vi "Autonomous Independent.vi"() -> ()   [LabVIEW 2012]
doc: "This VI is called when autonomous begins, and will automatically be terminated when autonomous ends. You can carry out timed or sensor driven robot movement independently without needing to return to the caller."
uses:
  Robot Global Data.vi
  Motors Values.vi
panel:
  out "Current Movement, for debugging":T1 {"Y Joystick Value" scale=1.0..-1.0; "X Joystick Value" scale=-1.0..1.0}
  in  "Array of robot movements":T2(array[cluster]) {"Y Joystick Value" scale=1.0..-1.0; "X Joystick Value" scale=-1.0..1.0}
  # "Be sure to right-click and choose Data Operations>>Make Current Value default if you want to save the array values with the VI"
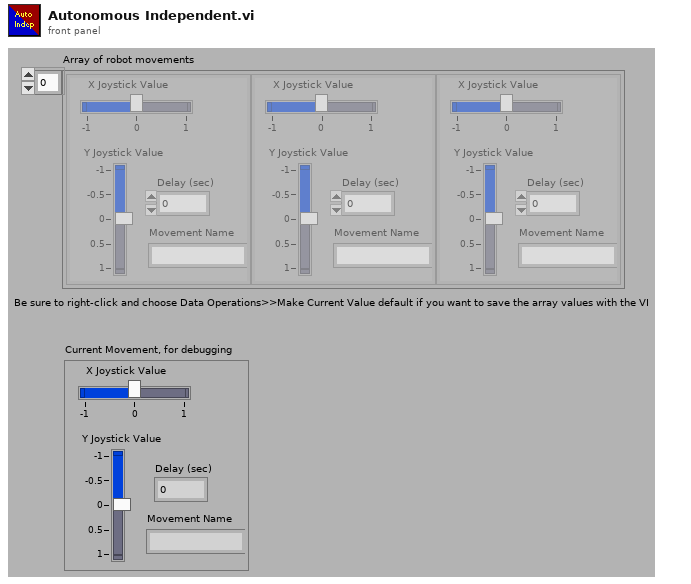
[diagram p1: front panel]
types:
  T1 = cluster{"X Joystick Value":dbl, "Y Joystick Value":dbl, "Delay (sec)":dbl, "Movement Name":string}
  T2 = cluster{"X Joystick Value":dbl, "Y Joystick Value":dbl, "Delay (sec)":dbl, "Movement Name":string}[]
  T3 = typedef "WPI_JoystickDevRef.ctl" = cluster{"Device":T4}
  T4 = typedef "WPI_JoystickDeviceEnum.ctl" = enum16{"USB 1", "USB 2", "USB 3", "USB 4", "Kinect 1", "Kinect 2"}
  T5 = typedef "WPI_DigitalInputDevRef.ctl" = cluster{"DevStatus":errorcluster, "DIO Channel":T6, "Digital Module":T7}
  T6 = typedef "FPGA_DIOChannel.ctl" = enum8{"DIO 1", "DIO 2", "DIO 3", "DIO 4", "DIO 5", "DIO 6", "DIO 7", "DIO 8", "DIO 9", "DIO 10", "DIO 11", "DIO 12", "DIO 13", "DIO 14", "Invalid"}
  T7 = typedef "FPGA_TypedefDigitalModule.ctl" = enum16{"Digital Module 1", "Digital Module 2"}
  T8 = typedef "WPI_RobotDriveDevRef.ctl" = cluster{"DevStatus":errorcluster, "Motors[]":T9[], "Square Inputs":bool, "Max Output":dbl, "Isochronous":bool}
  T9 = typedef "WPI_MotorControlDeviceRef.ctl" = cluster{"DeviceStatus":errorcluster, "Type":enum16{"PWM", "CAN"}, "PWM":cluster{"Digital Module":T7, "PWM Channel":T10, "DeadBand":T11}, "CAN":cluster{"Device Number":u8, "Control Mode":T12, "Semaphore":T13, "Max Vout":dbl}, "Invert":bool, "TransformRef":T14, "InvTransformRef":T14}
  T10 = typedef "FPGA_DIOPWMChannel.ctl" = enum8{"PWM 1", "PWM 2", "PWM 3", "PWM 4", "PWM 5", "PWM 6", "PWM 7", "PWM 8", "PWM 9", "PWM 10", "Invalid"}
  T11 = typedef "WPI_PWMDeadband.ctl" = cluster{"Name":string, "maxPositivePwm":i32, "minPositivePwm":i32, "centerPwm":i32, "maxNegativePwm":i32, "minNegativePwm":i32, "angularRange":u16}
  T12 = typedef "WPI_CANJaguar_ControlMode.ctl" = enum8{"Percent VBus", "Current", "Speed", "Position", "Voltage"}
  T13 = typedef "Semaphore RefNum" = refnum<k1>
  T14 = typedef "WPI_PWMTransform_ConPane.ctl" = refnum<vi>
  T15 = typedef "WPI_ServoDeviceRef.ctl" = cluster{"DeviceStatus":errorcluster, "Digital Module":T7, "PWM Channel":T10, "DeadBand":T11}
  T16 = cluster{"axis 1 (x)":dbl, "axis 2 (y)":dbl, "axis 3 (throttle)":dbl, "axis 4":dbl, "axis 5":dbl, "axis 6":dbl}
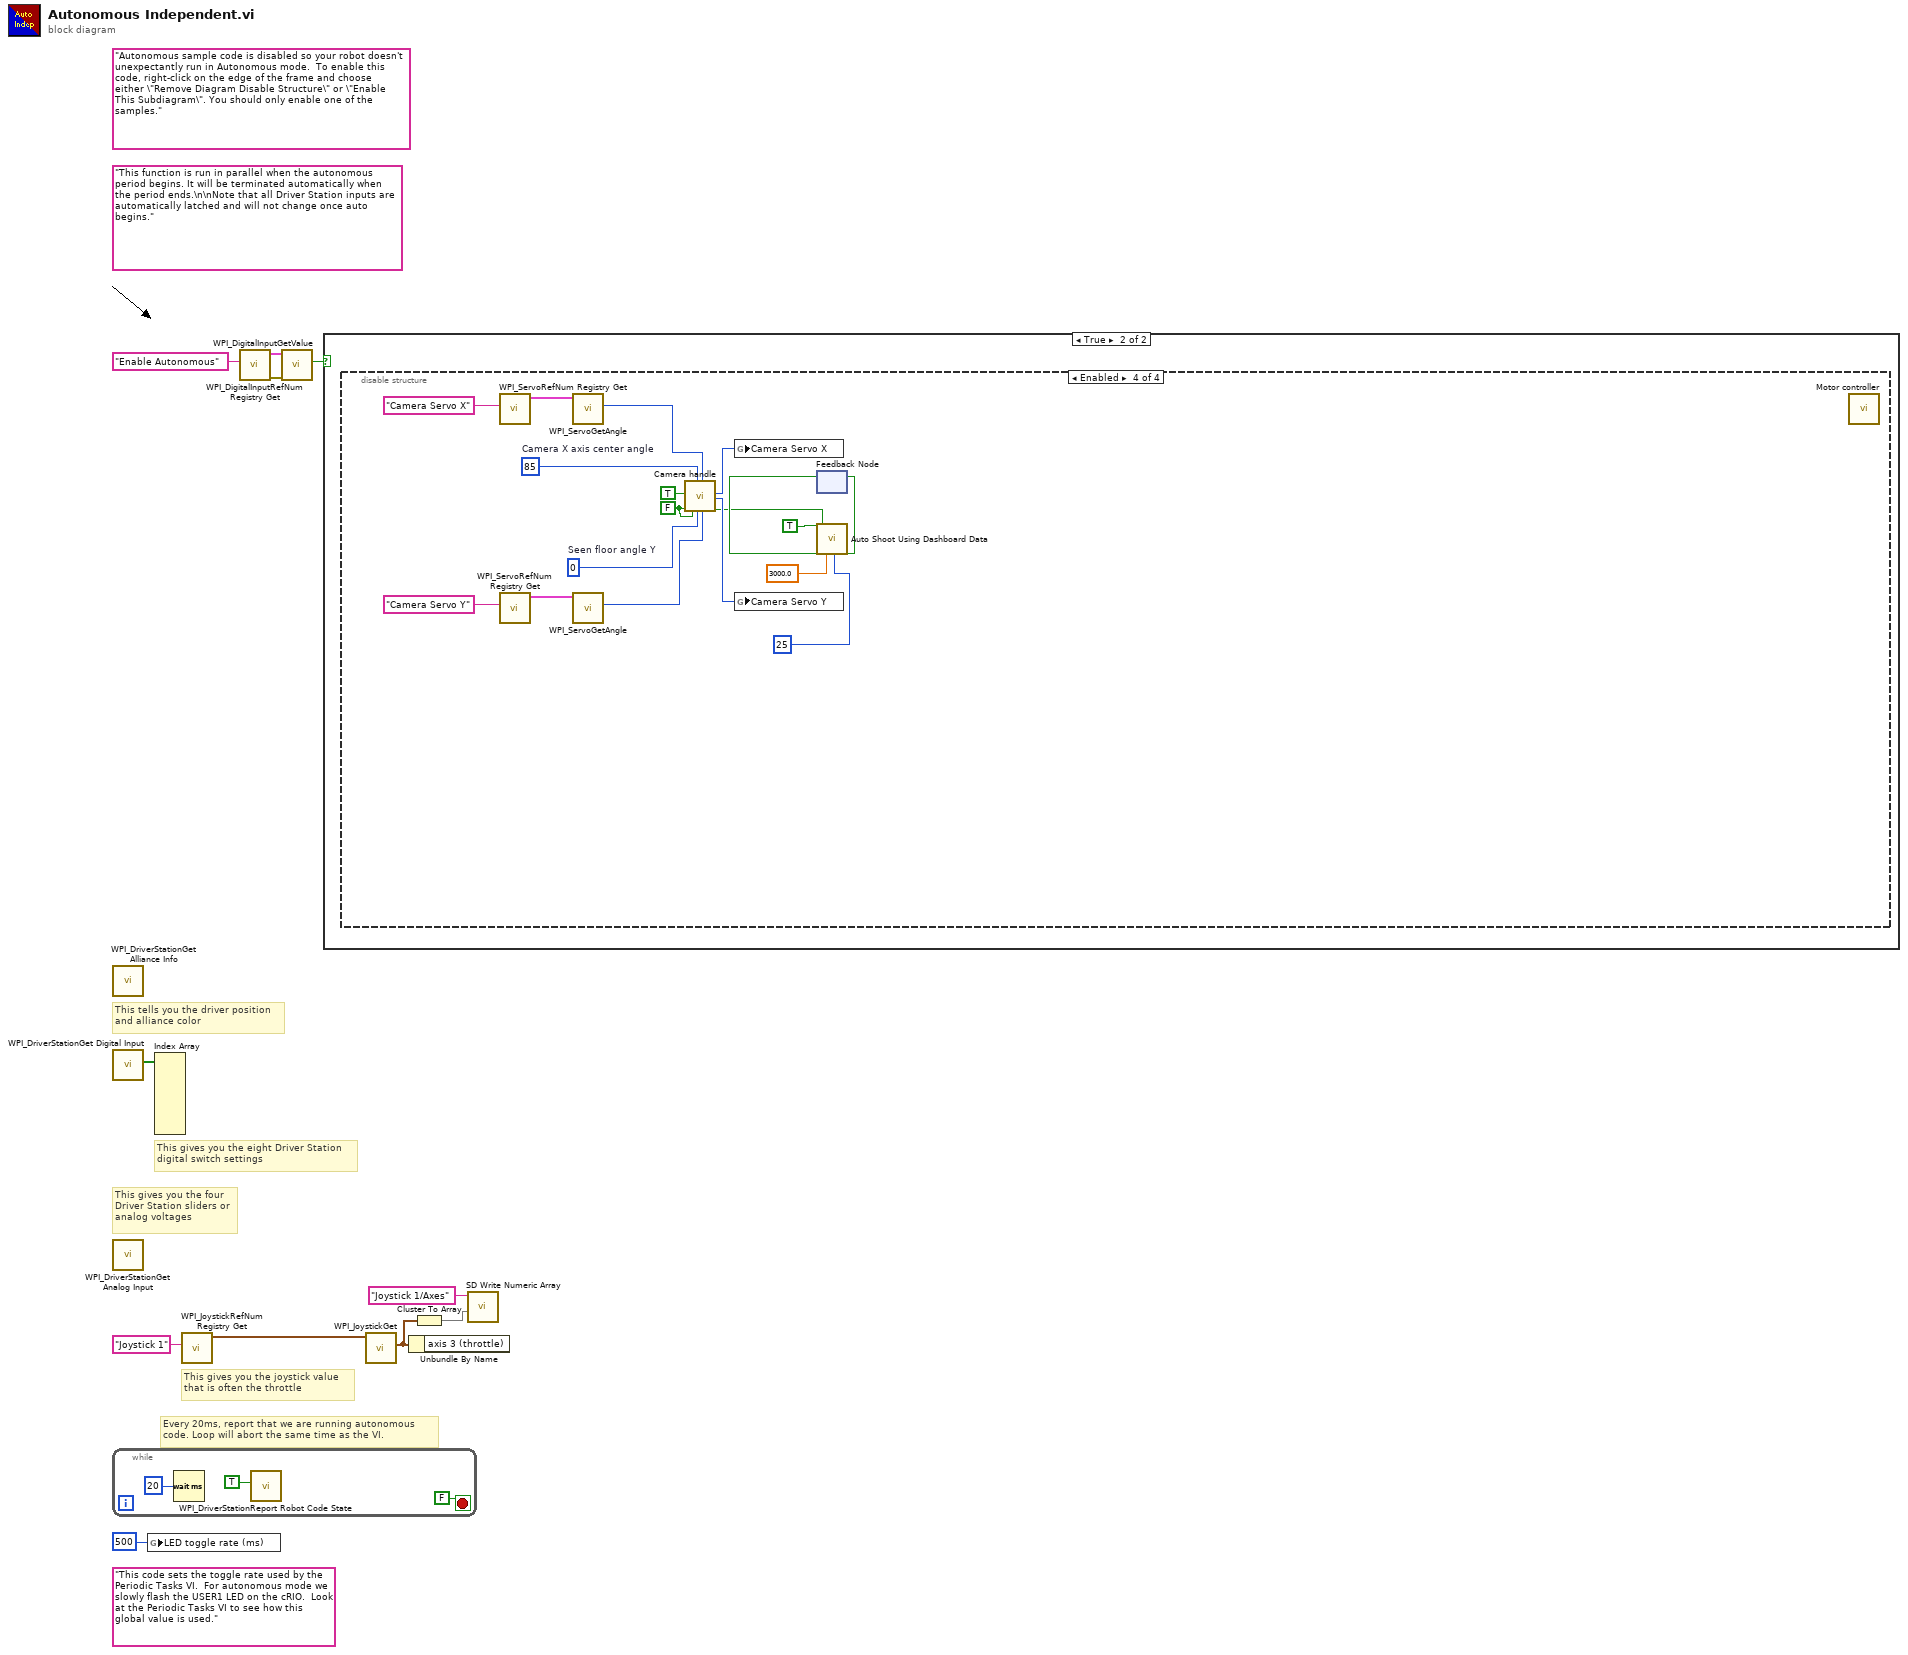
[diagram p0: block diagram]
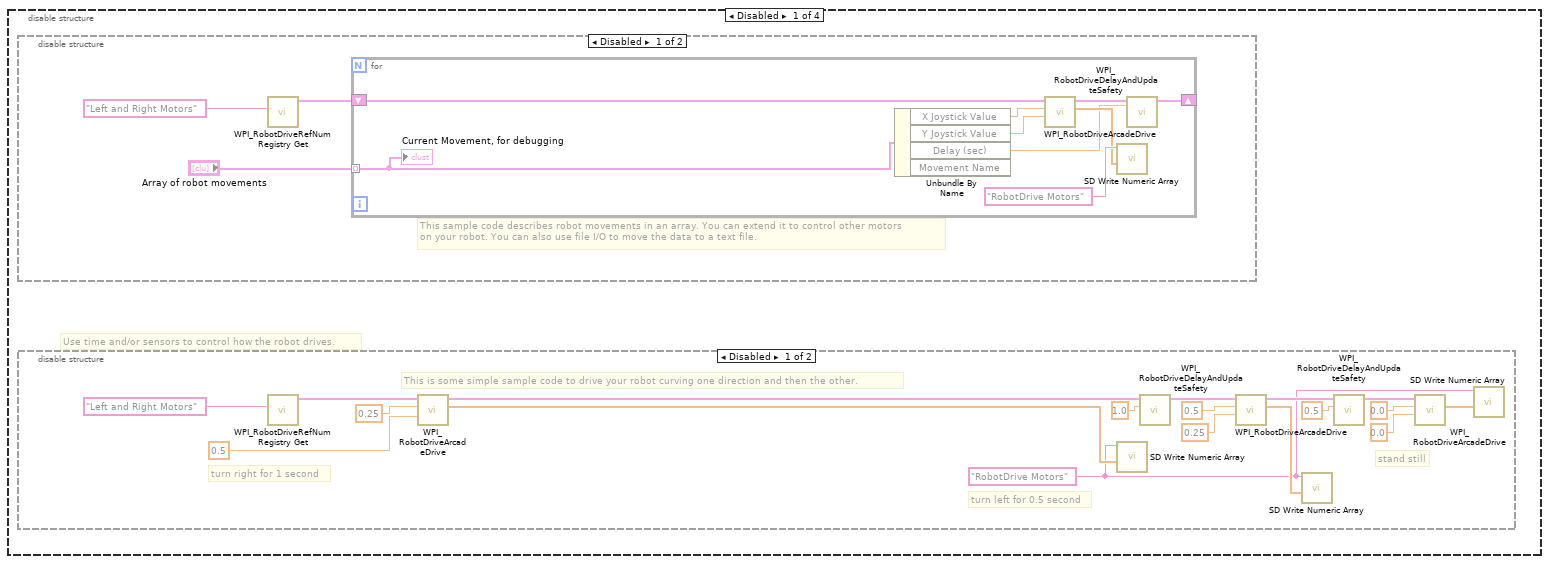
[diagram p3: hidden frame]
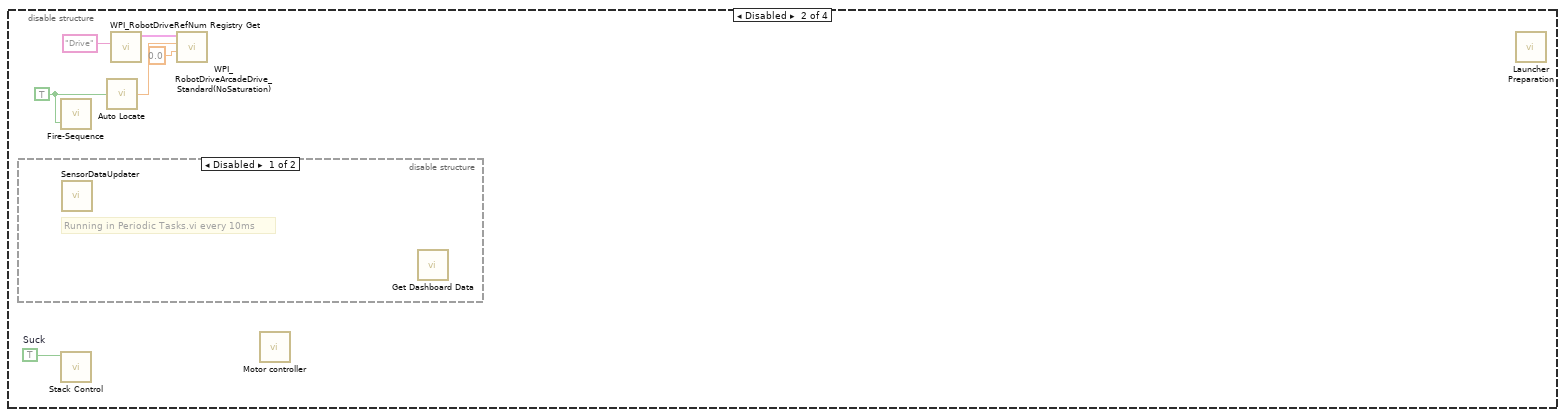
[diagram p6: hidden frame]
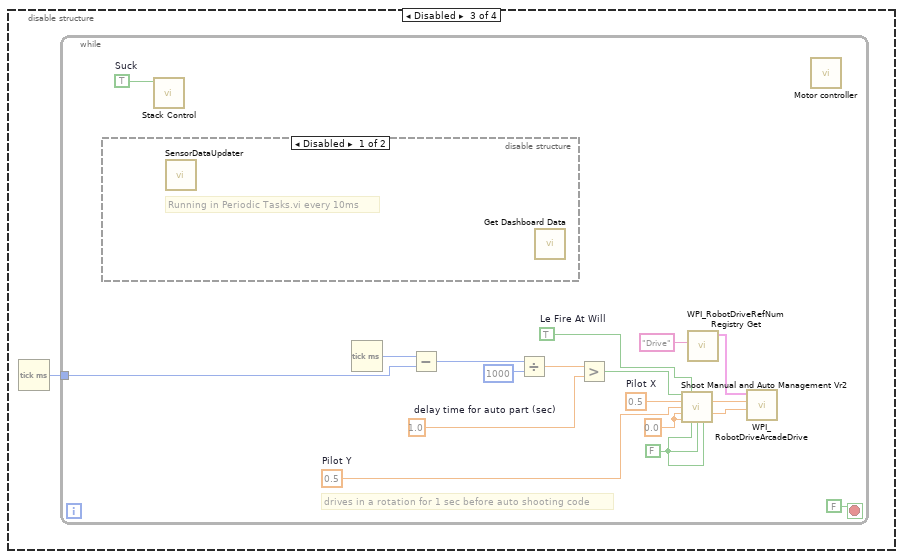
[diagram p8: hidden frame]
diagram:
  (unwired) "This code sets the toggle rate used by the Periodic Tasks VI.  For autonomous mode we slowly flash the USER1 LED on the cRIO.  Look at the Periodic Tasks VI to see how this global value is used."
  (unwired) "Autonomous sample code is disabled so your robot doesn't unexpectantly run in Autonomous mode.  To enable this code, right-click on the edge of the frame and choose either \"Remove Diagram Disable Structure\" or \"Enable This Subdiagram\". You should only enable one of the samples."
  (unwired) "This function is run in parallel when the autonomous period begins. It will be terminated automatically when the period ends.\n\nNote that all Driver Station inputs are automatically latched and will not change once auto begins."
  # "Every 20ms, report that we are running autonomous\ncode. Loop will abort the same time as the VI."
  # "This gives you the joystick value\nthat is often the throttle"
  # "This tells you the driver position\nand alliance color"
  # "This gives you the eight Driver Station\ndigital switch settings"
  # "This gives you the four\nDriver Station sliders or\nanalog voltages"
  n1 = call <vilib>:"WPI_DriverStationGet Alliance Info.vi"() -> ()  [unwired: 12 out]
  n2 = call <vilib>:"WPI_DriverStationGet Digital Input.vi"() -> ("Driver Station Digital Input (1-8)"=w11:bool[])  [unwired: 11 out]
  n3 = call <vilib>:"WPI_DriverStationGet Analog Input.vi"() -> ()  [unwired: 12 out]
  n4 = while {
    stop <- FALSE stop-if-true
    n5 = Wait (ms)(milliseconds to wait=u32 20) -> ()  [unwired: 1 out]
    n6 = call <vilib>:"WPI_DriverStationReport Robot Code State.vi"("Autonomous"=TRUE) -> ()  [unwired: 10 in, 1 out]
  }
  n7 = global write "Robot Global Data.vi" "LED toggle rate (ms)"(u32 500 ("LED ms toggle rate")) -> ()
  n8 = Index Array(array=w11) -> ()  [unwired: 8 in, 8 out]
  n9 = call <vilib>:"WPI_JoystickRefNum Registry Get.vi"("refnum name"="Joystick 1") -> ("JoystickDevRef"=w9:T3)  [unwired: 1 in, 9 out]
  n10 = call <vilib>:"WPI_DigitalInputRefNum Registry Get.vi"("refnum name"="Enable Autonomous") -> ("error out"=w2:errorcluster, "DigitalInputDevRef"=w4:T5)  [unwired: 9 in]
  n11 = call <vilib>:"WPI_DigitalInputGetValue.vi"("error in (no error)"=w2, "DigitalInputDevRef"=w4) -> ("Value"=w1:bool)  [unwired: 7 in, 2 out]
  n12 = case shown="True" w1 {
    frame False {
    }
    frame True {
      n13 = disable-structure shown="Enabled" {
        frame Disabled {
          # "Use time and/or sensors to control how the robot drives."
          n14 = disable-structure shown="Disabled" {
            frame Disabled {
              # "This sample code describes robot movements in an array. You can extend it to control other motors\non your robot. You can also use file I/O to move the data to a text file."
              n15 = call <vilib>:"WPI_RobotDriveRefNum Registry Get.vi"("refnum name"="Left and Right Motors") -> ("RobotDriveDevRef"=w16:T8)  [unwired: 1 in, 9 out]
              n16 = for {
                shift-right: [w22] -> _
                shift-left: w16 -> [w23]
                tunnel: "Array of robot movements" -> [w18] mode=indexing
                n17 = Unbundle By Name(w18) -> ("X Joystick Value"=w21:dbl, "Y Joystick Value"=w20:dbl, "Delay (sec)"=w19:dbl)  [unwired: 1 out]
                n18 = call-poly <vilib>:"WPI_RobotDriveArcadeDrive.vi"("Y axis value"=w20, "X axis value"=w21, "RobotDriveDevRef"=w23) -> ("Motor Values"=w25:dbl[], "RobotDriveDevRef"=w24:T8)  [unwired: 1 in, 6 out]
                n19 = call <vilib>:"SD Write Numeric Array.vi"("Numeric Array"=w25, "Name"="RobotDrive Motors") -> ()  [unwired: 8 in, 2 out]
                n20 = call <vilib>:"WPI_RobotDriveDelayAndUpdateSafety.vi"("Delay (s)"=w19, "RobotDriveDevRef"=w24) -> ("RobotDriveDevRef 2"=w22:T8)  [unwired: 8 in, 1 out]
                "Current Movement, for debugging" <- w18
              }
            }
            frame Enabled {
            }
          }
          n21 = disable-structure shown="Disabled" {
            frame Disabled {
              w27 = "RobotDrive Motors" ("Name")
              # "This is some simple sample code to drive your robot curving one direction and then the other."
              # "stand still"
              # "turn left for 0.5 second"
              # "turn right for 1 second"
              n22 = call <vilib>:"WPI_RobotDriveRefNum Registry Get.vi"("refnum name"="Left and Right Motors") -> ("RobotDriveDevRef"=w31:T8)  [unwired: 1 in, 9 out]
              n23 = call-poly <vilib>:"WPI_RobotDriveArcadeDrive.vi"("Y axis value"=0.5 ("X axis value"), "X axis value"=0.25, "RobotDriveDevRef"=w31) -> ("Motor Values"=w30:dbl[], "RobotDriveDevRef"=w38:T8)  [unwired: 1 in, 6 out]
              n24 = call <vilib>:"SD Write Numeric Array.vi"("Numeric Array"=w30, "Name"=w27) -> ()  [unwired: 8 in, 2 out]
              n25 = call <vilib>:"WPI_RobotDriveDelayAndUpdateSafety.vi"("Delay (s)"=1.0, "RobotDriveDevRef"=w38) -> ("RobotDriveDevRef 2"=w37:T8)  [unwired: 8 in, 1 out]
              n26 = call-poly <vilib>:"WPI_RobotDriveArcadeDrive.vi"("Y axis value"=0.25 ("X axis value"), "X axis value"=0.5, "RobotDriveDevRef"=w37) -> ("Motor Values"=w29:dbl[], "RobotDriveDevRef"=w36:T8)  [unwired: 1 in, 6 out]
              n27 = call <vilib>:"SD Write Numeric Array.vi"("Numeric Array"=w29, "Name"=w27) -> ()  [unwired: 8 in, 2 out]
              n28 = call <vilib>:"WPI_RobotDriveDelayAndUpdateSafety.vi"("Delay (s)"=0.5, "RobotDriveDevRef"=w36) -> ("RobotDriveDevRef 2"=w35:T8)  [unwired: 8 in, 1 out]
              n29 = call-poly <vilib>:"WPI_RobotDriveArcadeDrive.vi"("Y axis value"=0.0 ("X axis value"), "X axis value"=0.0, "RobotDriveDevRef"=w35) -> ("Motor Values"=w28:dbl[])  [unwired: 1 in, 7 out]
              n30 = call <vilib>:"SD Write Numeric Array.vi"("Numeric Array"=w28, "Name"=w27) -> ()  [unwired: 8 in, 2 out]
            }
            frame Enabled {
            }
          }
        }
        frame Disabled {
          w45 = TRUE  # Suck
          w47 = TRUE
          n31 = disable-structure shown="Disabled" {
            frame Disabled {
              # "Running in Periodic Tasks.vi every 10ms"
              n32 = call "SensorDataUpdater.vi"() -> ()  [unwired: 12 in]
              n33 = call "Get Dashboard Data.vi"() -> ()  [unwired: 12 in]
            }
            frame Enabled {
            }
          }
          n34 = call "Fire-Sequence.vi"("La Fire at will?"=w47) -> ()  [unwired: 3 in]
          n35 = call "Stack Control.vi"("Suck"=w45) -> ()  [unwired: 7 in, 4 out]
          n36 = call "Auto Locate.vi"("Autonomous?"=w47) -> ("X Drive Arcade"=w46:dbl)
          n37 = call <vilib>:"WPI_RobotDriveRefNum Registry Get.vi"("refnum name"="Drive") -> ("RobotDriveDevRef"=w49:T8)  [unwired: 1 in, 9 out]
          n38 = call <vilib>:"WPI_RobotDriveArcadeDrive_Standard(NoSaturation).vi"("Y axis value"=0.0, "X axis value"=w46, "RobotDriveDevRef"=w49) -> ()  [unwired: 1 in, 8 out]
          n39 = call "Motor controller.vi"() -> ()  [unwired: 12 in]
          n40 = call "Launcher Preparation.vi"() -> ()  [unwired: 5 in]
        }
        frame Disabled {
          n41 = Tick Count (ms)() -> (millisecond timer value=w51:u32)
          n42 = while {
            tunnel: w51 -> [w63]
            stop <- FALSE stop-if-true
            w52 = TRUE  # Suck
            w53 = FALSE
            w55 = 0.0 ("Elevation")
            w56 = 0.5  # Pilot Y
            w58 = 1.0  # delay time for auto part (sec)
            w60 = 0.5  # Pilot X
            w69 = TRUE  # Le Fire At Will
            # "drives in a rotation for 1 sec before auto shooting code"
            n43 = disable-structure shown="Disabled" {
              frame Disabled {
                # "Running in Periodic Tasks.vi every 10ms"
                n44 = call "SensorDataUpdater.vi"() -> ()  [unwired: 12 in]
                n45 = call "Get Dashboard Data.vi"() -> ()  [unwired: 12 in]
              }
              frame Enabled {
              }
            }
            n46 = call "Stack Control.vi"("Suck"=w52) -> ()  [unwired: 7 in, 4 out]
            n47 = Tick Count (ms)() -> (millisecond timer value=w64:u32)
            n48 = Subtract(x=w64, y=w63) -> (x-y=w62:u32)
            n49 = Divide(x=w62, y=u32 1000) -> (x/y=w59:dbl)
            n50 = Greater?(x=w59, y=w58) -> (0:w57:bool)
            n51 = call "Shoot Manual and Auto Management Vr2.vi"("Auto Preparation for Shooting"=w57, "Le Fire At Will"=w69, "Pilot X"=w60, "Pilot Y"=w56, "Elevation"=w55, "Shoot Motors"=w55, "Stop Centerizing"=w53, "ReCenterize"=w53, "Fine Tune"=w53) -> ("X Drive Arcade"=w67:dbl, "Y Drive Arcade"=w66:dbl)  [unwired: 4 in, 1 out]
            n52 = call <vilib>:"WPI_RobotDriveRefNum Registry Get.vi"("refnum name"="Drive") -> ("RobotDriveDevRef"=w65:T8)  [unwired: 9 in, 1 out]
            n53 = call-poly <vilib>:"WPI_RobotDriveArcadeDrive.vi"("Y axis value"=w66, "X axis value"=w67, "RobotDriveDevRef"=w65) -> ()  [unwired: 6 in, 3 out]
            n54 = call "Motor controller.vi"() -> ()  [unwired: 12 in]
          }
        }
        frame Enabled {
          w72 = FALSE ("View Ground")
          w84 = 85  # Camera X axis center angle
          w77 = 0  # Seen floor angle Y
          n55 = call <vilib>:"WPI_ServoRefNum Registry Get.vi"("refnum name"="Camera Servo X") -> ("ServoDeviceRef"=w83:T15)  [unwired: 9 in, 1 out]
          n56 = call <vilib>:"WPI_ServoRefNum Registry Get.vi"("refnum name"="Camera Servo Y") -> ("ServoDeviceRef"=w79:T15)  [unwired: 9 in, 1 out]
          n57 = call <vilib>:"WPI_ServoGetAngle.vi"("ServoDeviceRef"=w83) -> ("Angle"=w81:u16)  [unwired: 7 in, 2 out]
          n58 = call <vilib>:"WPI_ServoGetAngle.vi"("ServoDeviceRef"=w79) -> ("Angle"=w80:u16)  [unwired: 7 in, 2 out]
          n59 = call "Camera handle.vi"("Center on Target"=TRUE, "View Ground"=w72, "Stop Auto Cam movement"=w72, "Camera X axis center angle"=w84, "Seen floor angle Y"=w77, "Servo Get Angle X"=w81, "Servo Get Angle Y"=w80) -> ("Out X [angle]"=w76:i32, "Out Y [angle]"=w75:i32, "Camera Centered on Target"=w74:bool)  [unwired: 10 in]
          n60 = global write "Motors Values.vi" "Camera Servo X"(w76) -> ()
          n61 = global write "Motors Values.vi" "Camera Servo Y"(w75) -> ()
          n62 = feedback #1() -> (w86:bool)  [unwired: 1 in]
          n63 = call "Auto Shoot Using Dashboard Data.vi"("Auto Preparation for Shooting"=TRUE, "Le Fire At Will"=w86, "Camera Centered?"=w74, "Set Point RPM"=3000.0 ("Shoot Motors"), "Angle Set Point"=25) -> ("Ready to Fire!"=w87:bool)  [unwired: 20 in, 2 out]
          n64 = feedback-in #1(w87) -> ()
          n65 = call "Motor controller.vi"() -> ()  [unwired: 12 in]
        }
      }
    }
  }
  n66 = call <vilib>:"WPI_JoystickGet.vi"("JoystickDevRef"=w9) -> ("Axes"=w6:T16)  [unwired: 1 in, 5 out]
  n67 = Unbundle By Name(w6) -> ()  [unwired: 1 out]
  n68 = Cluster To Array(cluster=w6) -> (array=w7:dbl[])
  n69 = call <vilib>:"SD Write Numeric Array.vi"("Numeric Array"=w7, "Name"="Joystick 1/Axes") -> ()  [unwired: 8 in, 2 out]
